vi "PenaltyAttackerTactic.vi"(8 "error in (no error)":errorcluster, 9 "Game":refnum<class "Game.lvclass">, 10 "Robot":refnum<class "Robot.lvclass">, 11 "PenaltyAttackerTactic in":refnum<class "PenaltyAttackerTactic.lvclass">) -> (0 "error out":errorcluster, 2 "Robot out":refnum<class "Robot.lvclass">, 3 "PenaltyAttackerTactic out":refnum<class "PenaltyAttackerTactic.lvclass">)   [LabVIEW 2018, in "PenaltyAttackerTactic.lvclass"]
uses:
  PenaltyAttackerTactic.lvclass
  C:/Users/Gustavo/Desktop/RoboIME/SimplePass/SSL_AI/Tactic_class/Tactic.lvclass
  Robot_class/Robot.lvclass
  Game_class/Game.lvclass
  Tactic_class/Tactic.lvclass/Tactic.ctl
  Robot_class/tactics.ctl
  Skillbook_class/Skillbook.lvclass/Skillbook.ctl
  PenaltyAttackerTactic.lvclass/PenaltyAttackerTactic.ctl
  Robot_class/Robot.lvclass/Robot.ctl
  Skillbook_class/Read PenaltyAttackerSkill 1.vi
  Tactic_class/Read Skillbook.vi
  Robot_class/Write tactic.vi
  Write States.vi
  Skillbook_class/Skillbook.lvclass
  PenaltyAttackerSkill_class/PenaltyAttackerSkill.lvclass
panel:
  out "x .or. y?":bool
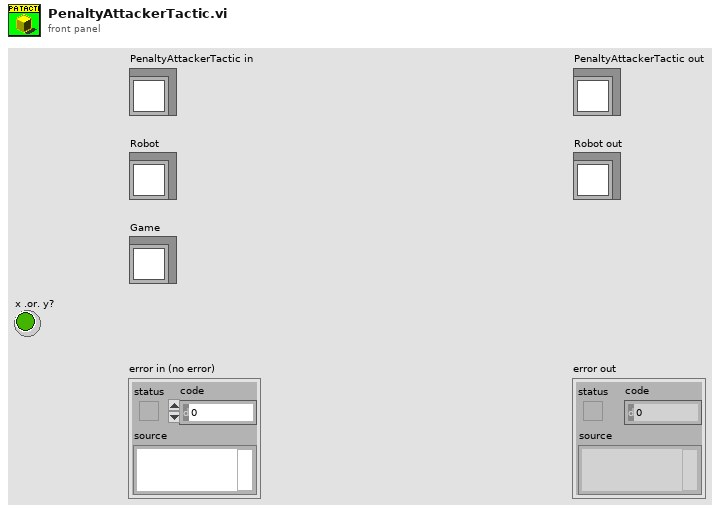
[diagram p1: front panel]
types:
  T1 = typedef "tactics.ctl" = enum16{"PenaltyAttacker", "PassObserver", "PenaltyDefense", "Test", "DefendGoal", "Marker", "FollowAttacker", "DefendArea", "Shoot", "AttackerAimGoal", "AttackerBallOutOfField", "AttackerBlock", "AttackerStop", "Duelist", "Halt", "ZigZag", "GoTo", "Timeout", "KickToPassReceiver", "PositionToReceivePass", "PassReceiver", "WaitPass"}
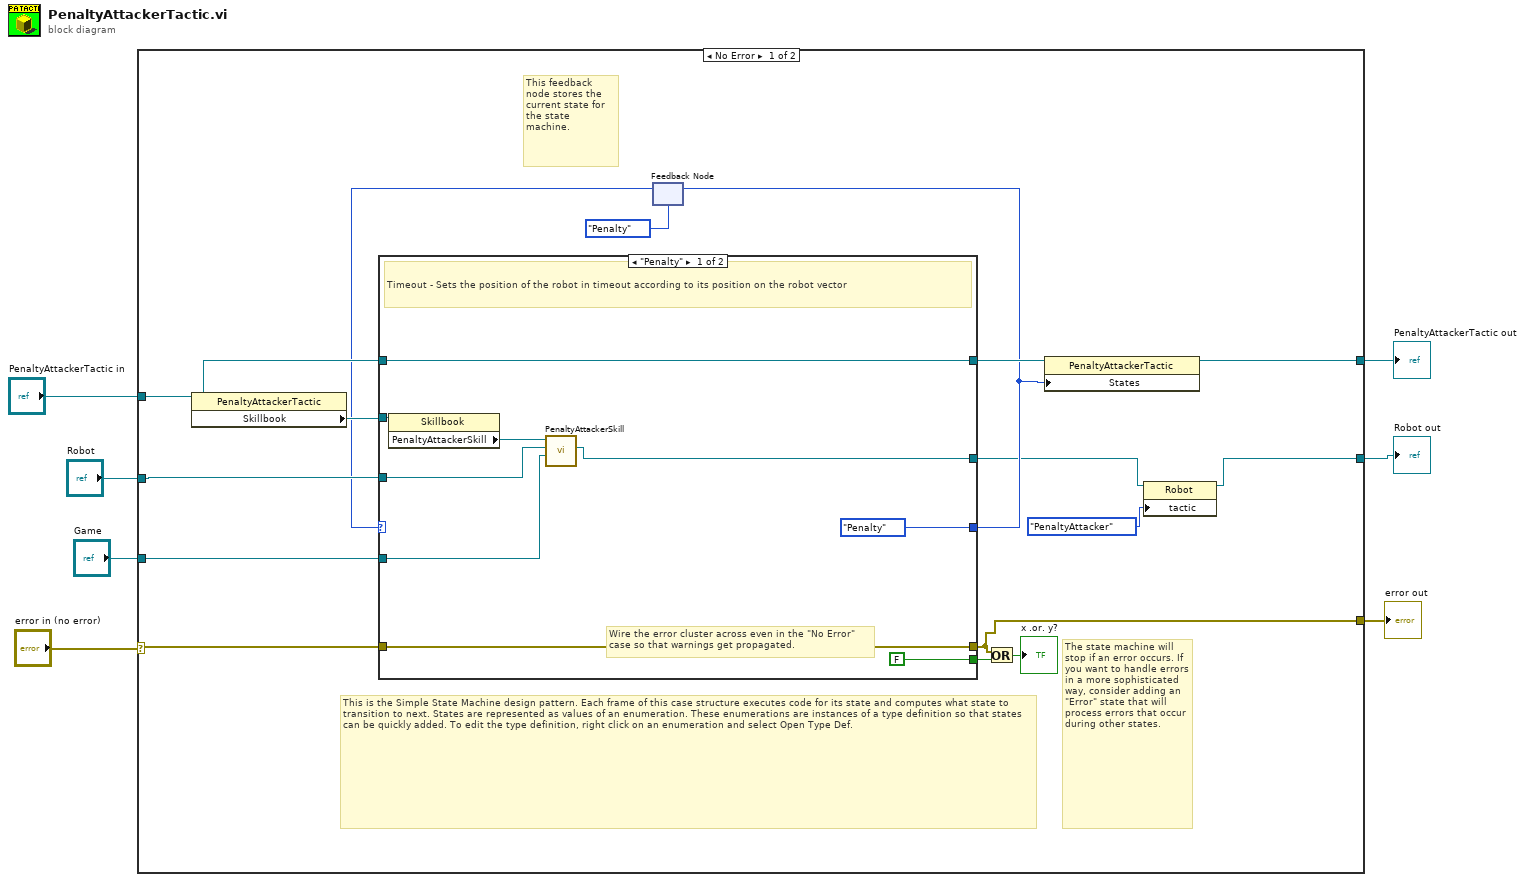
[diagram p0: block diagram]
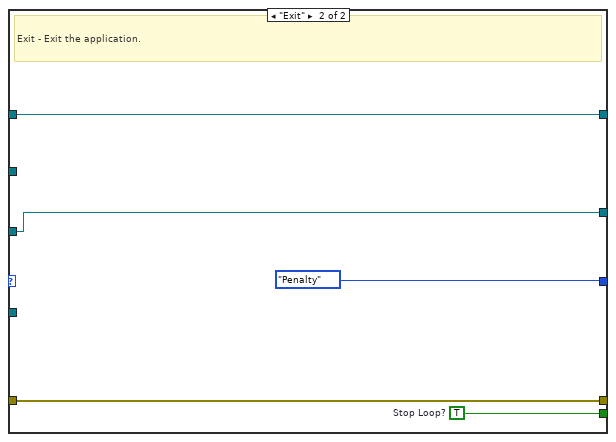
[diagram p2: hidden frame]
diagram:
  n1 = case shown="No Error" "error in (no error)" {
    selector: "error in (no error)" -> [w17 w40]
    tunnel: [w16 w40] -> w6
    tunnel: [w13 w39] -> w4
    tunnel: "PenaltyAttackerTactic in" -> [w19 w39]
    tunnel: "Robot" -> [w18 w38]
    tunnel: "Game" -> [w15 _]
    tunnel: [w8 w38] -> w1
    frame No Error {
      # "The state machine will stop if an error occurs. If you want to handle errors in a more sophisticated way, consider adding an \"Error\" state that will process errors that occur during other states."
      # "This feedback node stores the current state for the state machine."
      # "This is the Simple State Machine design pattern. Each frame of this case structure executes code for its state and computes what state to transition to next. States are represented as values of an enumeration. These enumerations are instances of a type definition so that states can be quickly added. To edit the type definition, right click on an enumeration and select Open Type Def."
      # "Wire the error cluster across even in the \"No Error\"\ncase so that warnings get propagated."
      n2 = property class="PenaltyAttackerTactic"(reference=w19) -> ("Skillbook"=w21:refnum<class "Skillbook.lvclass">)  [unwired: 1 in, 2 out]
      n3 = feedback #1(enum16{"Exit", "Penalty"}."Penalty" ("States")) -> (w11:enum16{"Exit", "Penalty"})
      n4 = case shown="\"Penalty\"" w11 {
        tunnel: [enum16{"Exit", "Penalty"}."Penalty" ("States") enum16{"Exit", "Penalty"}."Penalty" ("States")] -> w12
        tunnel: [FALSE ("Stop Loop?") w37] -> w23
        tunnel: w21 -> [w25 _]
        tunnel: [w30 w35] -> w9
        tunnel: [w31 w36] -> w20
        tunnel: w19 -> [w31 w36]
        tunnel: w18 -> [w29 w35]
        tunnel: [w28 w34] -> w16
        tunnel: w17 -> [w28 w34]
        tunnel: w15 -> [w26 _]
        frame "Penalty" {
          # "Timeout - Sets the position of the robot in timeout according to its position on the robot vector"
          n5 = property class="Skillbook"(reference=w25) -> ("PenaltyAttackerSkill"=w24:refnum<class "PenaltyAttackerSkill.lvclass">)  [unwired: 1 in, 2 out]
          n6 = call-dynamic "PenaltyAttackerSkill.vi"("Game"=w26, "Robot"=w29, "PenaltyAttackerSkill in"=w24) -> ("Robot out"=w30:refnum<class "Robot.lvclass">)  [unwired: 6 in, 2 out]
        }
        frame "Exit" {
          w37 = TRUE  # Stop Loop?
          # "Exit - Exit the application."
        }
      }
      n7 = feedback-in #1(w12) -> ()
      n8 = Or(x=w16, y=w23) -> (x .or. y?=→"x .or. y?":bool)
      n9 = property class="PenaltyAttackerTactic"(reference=w20, "States"=w12) -> (reference out=w13:refnum<class "PenaltyAttackerTactic.lvclass">)  [unwired: 1 in, 1 out]
      n10 = property class="Robot"(reference=w9, "tactic"=tactics."PenaltyAttacker") -> (reference out=w8:refnum<class "Robot.lvclass">)  [unwired: 1 in, 1 out]
    }
    frame Error {
    }
  }
  "error out" <- w6
  "PenaltyAttackerTactic out" <- w4
  "Robot out" <- w1
